vi "GFITS_LibClose.vi"(8 "error in (no error)":errorcluster) -> (0 "error out":errorcluster, 2 "return value":i32)   [LabVIEW 2016]
uses:
  c/lib/libgfits.so
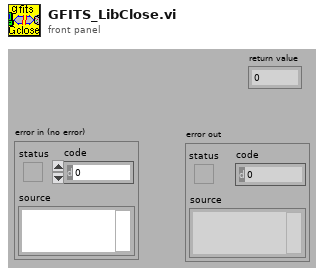
[diagram p1: front panel]
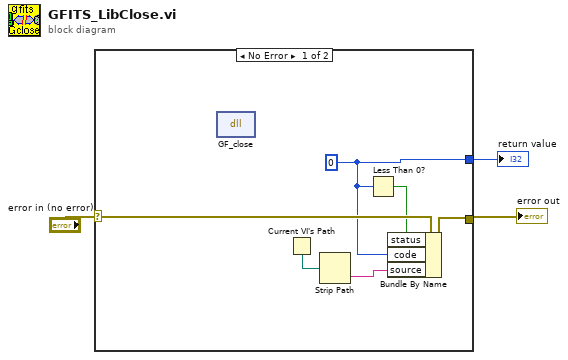
[diagram p0: block diagram]
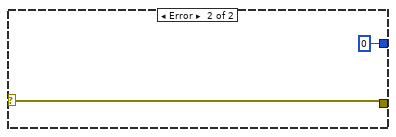
[diagram p2: hidden frame]
diagram:
  n1 = case shown="No Error" "error in (no error)" {
    selector: "error in (no error)" -> [w9 w11]
    tunnel: [w4 0] -> w3
    tunnel: [w5 w11] -> w1
    frame No Error {
      w4 = 0
      n2 = dll-call lib="home/simager/panview/PAN/Modules/GFITS/private/c/lib/libgfits.so" fn="GF_close"() -> ()  [unwired: 3 in, 3 out]
      n3 = Current VI's Path() -> (path=w7:path)
      n4 = Strip Path(path=w7) -> (name=w6:string)  [unwired: 1 out]
      n5 = Less Than 0?(x=w4) -> (x < 0?=w8:bool)
      n6 = Bundle By Name(cluster=w9, "status"=w8, "code"=w4, "source"=w6) -> (w5:errorcluster)
    }
    frame Error {
    }
  }
  "return value" <- w3
  "error out" <- w1
